vi "AutoFeedForward.vi"(1 "Target Velocity (in/s)":dbl) -> (0 "Equivalent Joystick Command":dbl)   [LabVIEW 2019]
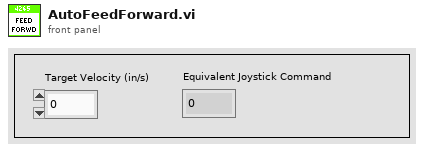
[diagram p1: front panel]
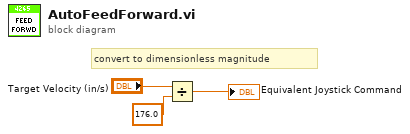
[diagram p0: block diagram]
diagram:
  # "convert to dimensionless magnitude"
  n1 = Divide(x="Target Velocity (in/s)", y=176.0) -> (x/y=→"Equivalent Joystick Command":dbl)
